vi "Write.vi"(8 "error in":errorcluster, 11 "server in":refnum<class "RT FlexRIO Server TCP.lvclass">) -> (0 "error out":errorcluster, 3 "server out":refnum<class "RT FlexRIO Server TCP.lvclass">)   [LabVIEW 2017, in "RT FlexRIO Server TCP.lvclass"]
uses:
  RT FlexRIO Server TCP.lvclass
  Properties/State_GET.vi
  Properties/Connection_GET.vi
  Properties/OutgoingQueue_GET.vi
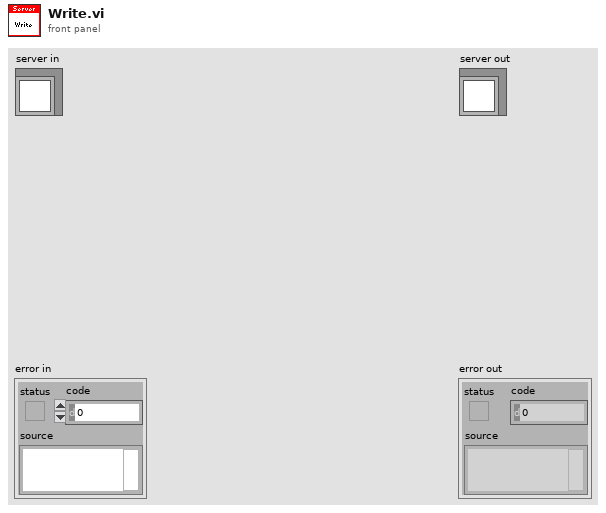
[diagram p1: front panel]
types:
  T1 = typedef "RT FlexRIO Server TCP.lvclass/State.ctl" = enum16{"started", "connected", "stopped"}
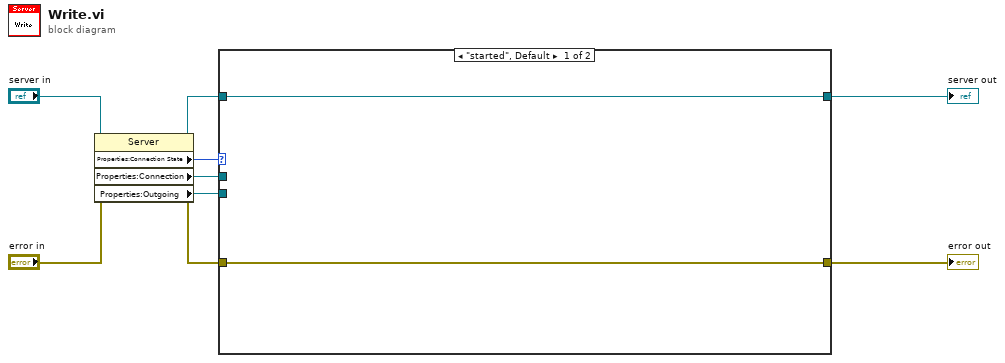
[diagram p0: block diagram]
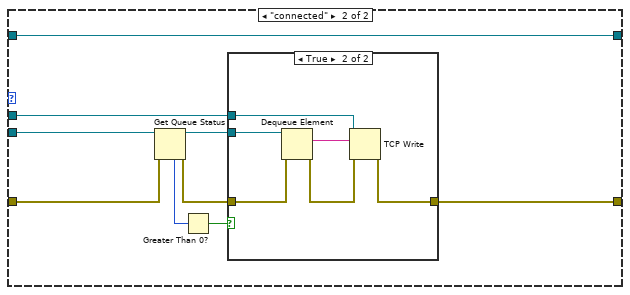
[diagram p2: hidden frame]
diagram:
  n1 = property class="Server"(reference="server in", error in="error in") -> (reference out=w4:refnum<class "RT FlexRIO Server TCP.lvclass">, error out=w3:errorcluster, "Properties:Connection State"=w5:T1, "Properties:Connection"=w2:refnum<k5>, "Properties:Outgoing"=w1:refnum<queue>)
  n2 = case shown="\"started\", Default" w5 {
    tunnel: w4 -> [w11 w16]
    tunnel: [w10 w17] -> w6
    tunnel: [w11 w16] -> w8
    tunnel: w3 -> [w10 w20]
    tunnel: w2 -> [_ w18]
    tunnel: w1 -> [_ w19]
    frame "started", Default {
    }
    frame "connected" {
      n3 = Get Queue Status(queue=w19, error in (no error)=w20) -> (queue out=w15:refnum<queue>, error out=w14:errorcluster, # elements in queue=w13:i32)  [unwired: 1 in, 5 out]
      n4 = Greater Than 0?(x=w13) -> (x > 0?=w12:bool)
      n5 = case shown="True" w12 {
        tunnel: w18 -> [_ w24]
        tunnel: [w21 w22] -> w17
        tunnel: w15 -> [_ w27]
        tunnel: w14 -> [w21 w26]
        frame False {
        }
        frame True {
          n6 = Dequeue Element(queue=w27, error in (no error)=w26) -> (element=w25:string, error out=w23:errorcluster)  [unwired: 1 in, 2 out]
          n7 = TCP Write(connection ID=w24, data in=w25, error in (no error)=w23) -> (error out=w22:errorcluster)  [unwired: 1 in, 2 out]
        }
      }
    }
  }
  "error out" <- w6
  "server out" <- w8
